vi "Display Name to Datafinder Field name.vi"(8 "error in (no error)":errorcluster, 9 "eSearch Type In":T1, 10 "Field Display Name":string, 11 "Connection Refnum":T2) -> (0 "error out":errorcluster, 1 "eSearch Type Out":T1, 2 "Datafinder Search Name":string, 3 "Connection Refnum Out":T2)   [LabVIEW 2011]
uses:
  SI.LIB/ODBC/SQL Controls/Connection Refnum.ctl
  eSearch Types.ctl
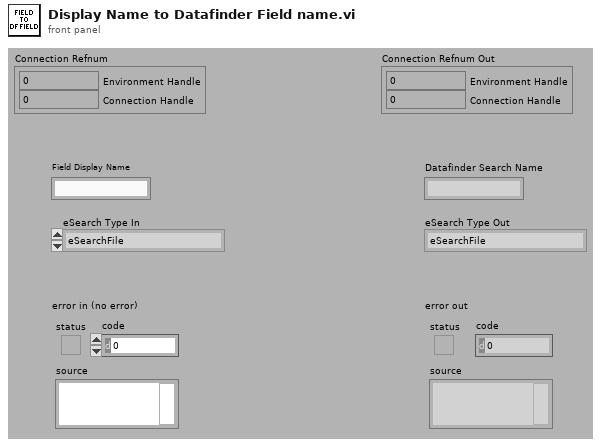
[diagram p1: front panel]
types:
  T1 = typedef "eSearch Types.ctl" = enum16{"eSearchFile", "eSearchChannelGroup", "eSearchChannel"}
  T2 = typedef "Connection Refnum.ctl" = cluster{"Environment Handle":i32, "Connection Handle":i32}
  T3 = typedef "Field Record.ctl" = cluster{"ixField":i32, "iSequenceOrder":i32, "sxFieldId":string, "sxSequenceId":string, "sDisplayName":string, "sValue":string, "sUnits":string, "nDataType":T4, "nNextItem":T5, "fSystem":bool, "fSystemValue":bool, "fRequired":bool, "fSetAtTest":bool, "fTestField":bool, "fDeleted":bool, "fIndexed":bool, "fFreeList":bool}
  T4 = typedef "Field DataTypes.ctl" = enum32{"text", "numeric", "list", "timestamp", "boolean"}
  T5 = typedef "Field NextItem.ctl" = enum32{"Reset", "Retain", "Auto-Increment"}
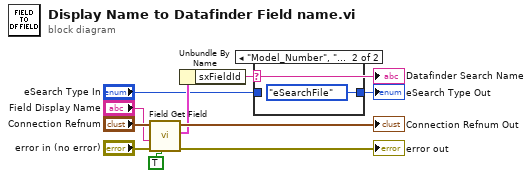
[diagram p0: block diagram]
diagram:
  n1 = call "Field Get Field.vi"("by sDisplayName? (f, by sFieldId)"=TRUE, "error in (no error)"="error in (no error)", "sFieldId or sDisplayName (\"\")"="Field Display Name", "Connection Refnum"="Connection Refnum") -> ("error out"=→"error out":errorcluster, "Field"=w5:T3, "Connection Refnum"=→"Connection Refnum Out":T2)  [unwired: 1 in, 4 out]
  n2 = Unbundle By Name(w5) -> ("sxFieldId"=w2:string)
  "Datafinder Search Name" <- w2
  n3 = case shown="\"Model_Number\", \"Serial_Number\", \"Test_Type\"" w2 {
    tunnel: "eSearch Type In" -> [w11 _]
    tunnel: [w11 eSearch_Types."eSearchFile" ("eSearch Type In")] -> w3
    frame Default {
    }
    frame "Model_Number", "Serial_Number", "Test_Type" {
    }
  }
  "eSearch Type Out" <- w3
